vi "Create reply queue name (SubVI).vi"(1 "Correlation ID":string) -> (0 "reply queue name":string)   [LabVIEW 2016]
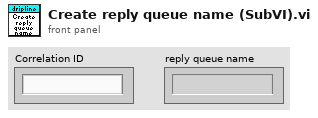
[diagram p1: front panel]
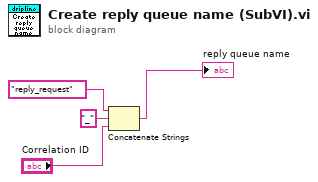
[diagram p0: block diagram]
diagram:
  n1 = Concatenate Strings("reply_request", "_" ("string"), "Correlation ID") -> (→"reply queue name":string)
